vi "Engine-Render.vi"(8 "error in (no error)":errorcluster, 11 "GLF Window in":refnum<class "Window.lvclass">) -> (0 "error out":errorcluster, 3 "GLF Window out":refnum<class "Window.lvclass">)   [LabVIEW 2020, in "GLF.lvlib" / "Window.lvclass"]
uses:
  Window.lvclass
  Window.lvclass/Window.ctl
  IAmVIEW/IAmVIEW.lvclass
  <vilib>/Saukko/LV SDL3/Sources/SDL3/Render/Render.lvlib
  <vilib>/Saukko/LV SDL3/Sources/SDL3/Video/Video.lvlib
  <vilib>/Saukko/LV SDL3/Sources/SDL3/Video/WindowFlags--ring.ctl
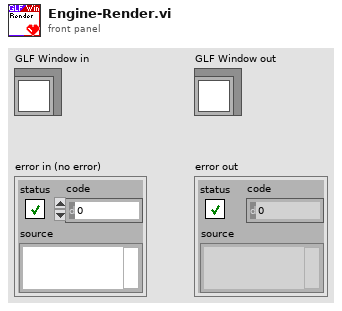
[diagram p1: front panel]
types:
  T1 = typedef "SDL3.lvlib/Video.lvlib/WindowFlags--ring.ctl" = u64
  T2 = typedef "GLF.lvlib/Window.lvclass/DVR--cluster.ctl" = cluster{"SDL_Window *":T3, "Window ID":T4, "SDL_Renderer *":T5, "Event Interface":refnum<class "WindowEventInterface.lvclass">, "VIEW":refnum<class "IAmVIEW.lvclass">, "Flags":T6}
  T3 = typedef "SDL3.lvlib/Video.lvlib/SDL_Window--pointer.ctl" = i64
  T4 = typedef "SDL3.lvlib/Video.lvlib/WindowID--integer.ctl" = u32
  T5 = typedef "SDL3.lvlib/Render.lvlib/SDL_Renderer--pointer.ctl" = i64
  T6 = typedef "GLF.lvlib/Window.lvclass/Flags--cluster.ctl" = cluster{"VIEW Needs Render":bool}
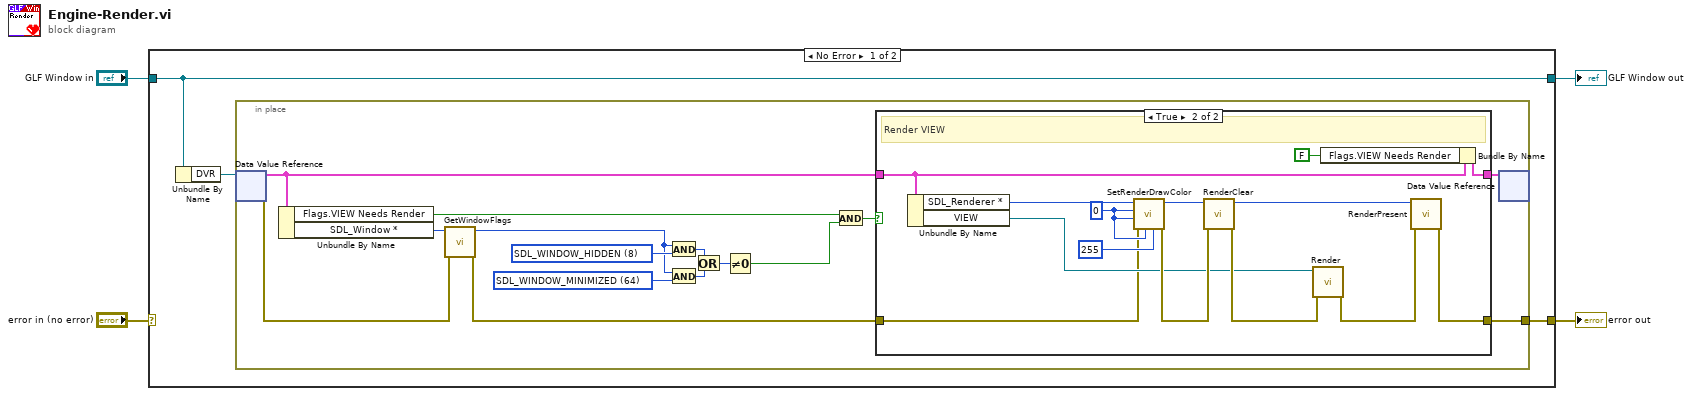
[diagram p0: block diagram]
diagram:
  n1 = case shown="No Error" "error in (no error)" {
    selector: "error in (no error)" -> [_ w38]
    tunnel: [w5 w38] -> w3
    tunnel: [w7 w37] -> w1
    tunnel: "GLF Window in" -> [w7 w37]
    frame No Error {
      n2 = Unbundle By Name(w7) -> ("DVR"=w6:refnum<data-value>)
      n3 = in-place {
        in-place-border: [w20] -> w5
        w13 = T1 8 items=["0"=0, "SDL_WINDOW_FULLSCREEN"=1, "SDL_WINDOW_OPENGL"=2, "SDL_WINDOW_OCCLUDED"=4, "SDL_WINDOW_HIDDEN"=8, "SDL_WINDOW_BORDERLESS"=16, "SDL_WINDOW_RESIZABLE"=32, "SDL_WINDOW_MINIMIZED"=64, "SDL_WINDOW_MAXIMIZED"=128, "SDL_WINDOW_MOUSE_GRABBED"=256, "SDL_WINDOW_INPUT_FOCUS"=512, "SDL_WINDOW_MOUSE_FOCUS"=1024, "SDL_WINDOW_EXTERNAL"=2048, "SDL_WINDOW_MODAL"=4096, "SDL_WINDOW_HIGH_PIXEL_DENSITY"=8192, "SDL_WINDOW_MOUSE_CAPTURE"=16384, "SDL_WINDOW_MOUSE_RELATIVE_MODE"=32768, "SDL_WINDOW_ALWAYS_ON_TOP"=65536, "SDL_WINDOW_UTILITY"=131072, "SDL_WINDOW_TOOLTIP"=262144, "SDL_WINDOW_POPUP_MENU"=524288, "SDL_WINDOW_KEYBOARD_GRABBED"=1048576, "SDL_WINDOW_VULKAN"=268435456, "SDL_WINDOW_METAL"=536870912, "SDL_WINDOW_TRANSPARENT"=1073741824, "SDL_WINDOW_NOT_FOCUSABLE"=2147483648] ("Window Flags")
        w15 = T1 64 items=["0"=0, "SDL_WINDOW_FULLSCREEN"=1, "SDL_WINDOW_OPENGL"=2, "SDL_WINDOW_OCCLUDED"=4, "SDL_WINDOW_HIDDEN"=8, "SDL_WINDOW_BORDERLESS"=16, "SDL_WINDOW_RESIZABLE"=32, "SDL_WINDOW_MINIMIZED"=64, "SDL_WINDOW_MAXIMIZED"=128, "SDL_WINDOW_MOUSE_GRABBED"=256, "SDL_WINDOW_INPUT_FOCUS"=512, "SDL_WINDOW_MOUSE_FOCUS"=1024, "SDL_WINDOW_EXTERNAL"=2048, "SDL_WINDOW_MODAL"=4096, "SDL_WINDOW_HIGH_PIXEL_DENSITY"=8192, "SDL_WINDOW_MOUSE_CAPTURE"=16384, "SDL_WINDOW_MOUSE_RELATIVE_MODE"=32768, "SDL_WINDOW_ALWAYS_ON_TOP"=65536, "SDL_WINDOW_UTILITY"=131072, "SDL_WINDOW_TOOLTIP"=262144, "SDL_WINDOW_POPUP_MENU"=524288, "SDL_WINDOW_KEYBOARD_GRABBED"=1048576, "SDL_WINDOW_VULKAN"=268435456, "SDL_WINDOW_METAL"=536870912, "SDL_WINDOW_TRANSPARENT"=1073741824, "SDL_WINDOW_NOT_FOCUSABLE"=2147483648] ("Window Flags")
        n4 = in-place-dvr #1(w6) -> (w16:T2, w18:errorcluster)
        n5 = Unbundle By Name(w16) -> ("Flags.VIEW Needs Render"=w22:bool, "SDL_Window *"=w14:T3)
        n6 = call <vilib>:"GetWindowFlags.vi"("No Error"=w18, "Window [SDL_Window *]"=w14) -> ("Error Out"=w17:errorcluster, "Window Flags"=w12:T1)  [unwired: 8 in]
        n7 = And(x=w12, y=w13) -> (x .and. y?=w11:T1)
        n8 = And(x=w12, y=w15) -> (x .and. y?=w10:T1)
        n9 = Or(x=w11, y=w10) -> (x .or. y?=w9:T1)
        n10 = Not Equal To 0?(x=w9) -> (x != 0?=w8:bool)
        n11 = And(x=w22, y=w8) -> (x .and. y?=w19:bool)
        n12 = case shown="True" w19 {
          tunnel: [w23 w36] -> w20
          tunnel: w17 -> [w23 w25]
          tunnel: w16 -> [w24 w30]
          tunnel: [w24 w27] -> w21
          frame False {
            # "Don't render VIEW"
          }
          frame True {
            w34 = u8 0 ("r")
            # "Render VIEW"
            n13 = Unbundle By Name(w30) -> ("SDL_Renderer *"=w29:T5, "VIEW"=w28:refnum<class "IAmVIEW.lvclass">)
            n14 = call <vilib>:"SetRenderDrawColor.vi"("a"=u8 255, "b"=w34, "No Error"=w25, "g"=w34, "r"=w34, "Renderer [SDL_Renderer *]"=w29) -> ("error out"=w35:errorcluster)  [unwired: 5 in]
            n15 = call <vilib>:"RenderClear.vi"("No Error"=w35, "Renderer [SDL_Renderer *]"=w29) -> ("error out"=w32:errorcluster)  [unwired: 9 in]
            n16 = call-dynamic "Render.vi"("error in (no error)"=w32, "IAmVIEW in"=w28) -> ("error out"=w31:errorcluster)  [unwired: 9 in]
            n17 = Bundle By Name(cluster=w30, "Flags.VIEW Needs Render"=FALSE) -> (w27:T2)
            n18 = call <vilib>:"RenderPresent.vi"("No Error"=w31, "Renderer [SDL_Renderer *]"=w29) -> ("error out"=w36:errorcluster)  [unwired: 9 in]
          }
        }
        n19 = in-place-dvr #1(w21) -> ()  [unwired: 2 out]
      }
    }
    frame Error {
    }
  }
  "error out" <- w3
  "GLF Window out" <- w1
